vi "Write Units.vi"(8 "error in (no error)":errorcluster, 10 "Units":string, 11 "Tag in":refnum<class "Tag.lvclass">) -> (0 "error out":errorcluster, 3 "Tag out":refnum<class "Tag.lvclass">)   [LabVIEW 2020, in "Tag Engine Core.lvlib" / "Tag.lvclass"]
doc: "_SubVI_"
uses:
  Tag.lvclass
  Tag.lvclass/Tag.ctl
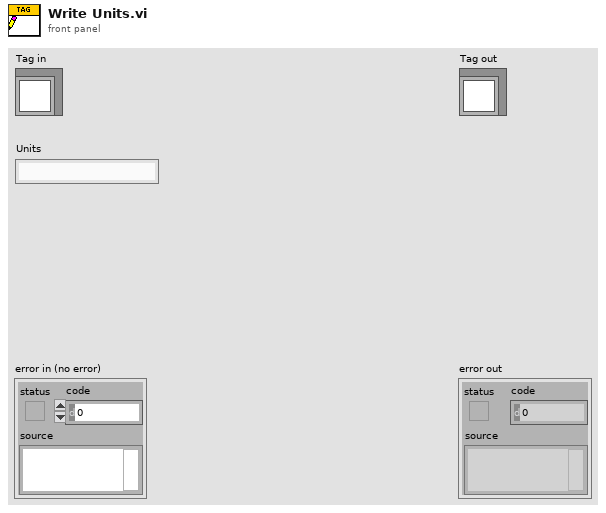
[diagram p1: front panel]
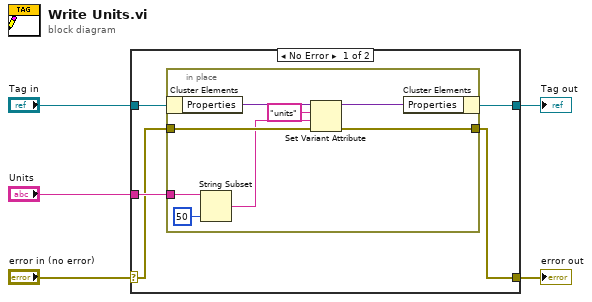
[diagram p0: block diagram]
diagram:
  n1 = case shown="No Error" "error in (no error)" {
    selector: "error in (no error)" -> [w8 w19]
    tunnel: [w7 w19] -> w4
    tunnel: [w6 w20] -> w2
    tunnel: "Tag in" -> [w10 w20]
    tunnel: "Units" -> [w9 _]
    frame No Error {
      n2 = in-place {
        in-place-border: w9 -> [w13]
        in-place-border: w8 -> [w15]
        in-place-border: [w14] -> w7
        n3 = in-place-cluster #1(w10) -> ("Properties"=w18:variant)
        n4 = String Subset(string=w13, length (rest)=50 ("length (rest)")) -> (substring=w12:string)  [unwired: 1 in]
        n5 = Set Variant Attribute(Variant=w18, name="units", value=w12, error in=w15) -> (Variant out=w16:variant, error out=w14:errorcluster)  [unwired: 1 out]
        n6 = in-place-cluster #1("Properties"=w16) -> (w6:refnum<class "Tag.lvclass">)
      }
    }
    frame Error {
    }
  }
  "error out" <- w4
  "Tag out" <- w2
